vi "Analog Output.vi"(10 "Voltage":dbl min=0.0 max=5.0, 11 "AO Channel":T1) -> ()   [LabVIEW 2016, in "navX Library.lvlib"]
uses:
  <vilib>/Rock Robotics/WPI/AnalogOutput/WPI_AnalogOutputChannel.ctl
  navX Library.lvlib
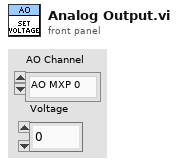
[diagram p1: front panel]
types:
  T1 = typedef "WPI_AnalogOutputChannel.ctl" = enum8{"AO MXP 0", "AO MXP 1", "Invalid"}
  T2 = typedef "WPI_AOChannelDevRef.ctl" = cluster{"DevStatus":errorcluster, "AO Channel":T1}
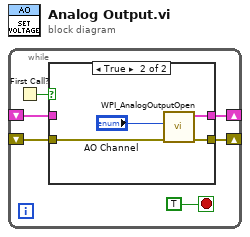
[diagram p0: block diagram]
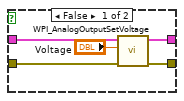
[diagram p2: hidden frame]
diagram:
  n1 = while {
    shift-right: [w5] -> _
    shift-left: _ -> [w4]
    shift-right: [w3] -> _
    shift-left: _ -> [w2]
    stop <- TRUE stop-if-true
    n2 = First Call?() -> (First Call?: T/F=w6:bool)
    n3 = case shown="True" w6 {
      tunnel: [w9 w15] -> w5
      tunnel: w4 -> [w11 w14]
      tunnel: [w10 w13] -> w3
      tunnel: w2 -> [w8 _]
      frame False {
        n4 = call <vilib>:"WPI_AnalogOutputSetVoltage.vi"("error in (no error)"=w11, "Voltage"="Voltage", "AODeviceRef"=w8) -> ("error out"=w9:errorcluster, "AODeviceRef"=w10:T2)  [unwired: 7 in]
      }
      frame True {
        n5 = call <vilib>:"WPI_AnalogOutputOpen.vi"("error in (no error)"=w14, "AO Channel"="AO Channel") -> ("error out"=w15:errorcluster, "AODeviceRef"=w13:T2)  [unwired: 8 in]
      }
    }
  }
